vi "Set Poses.vi"(8 "error in (no error)":errorcluster, 10 "serial arm poses":T1[](array[typedef]), 11 "serial arm in":refnum<class "NI_Robotics_Serial Robot Arm.lvclass">) -> (0 "error out":errorcluster, 3 "serial arm out":refnum<class "NI_Robotics_Serial Robot Arm.lvclass">)   [LabVIEW 2017, in "NI_Robotics_Serial Robot Arm.lvclass"]
doc: "Sets the joint angles that make up <B>serial arm poses</B> you want to associate with a robotic arm."
uses:
  <vilib>/robotics/Kinematics/Robot/NI_Robotics_Serial Robot Arm.lvclass
  <vilib>/robotics/Kinematics/Robot/Robot Pose.ctl
  <vilib>/robotics/Kinematics/Robot/NI_Robotics_Serial Robot Arm.lvclass/NI_Robotics_Serial Robot Arm.ctl
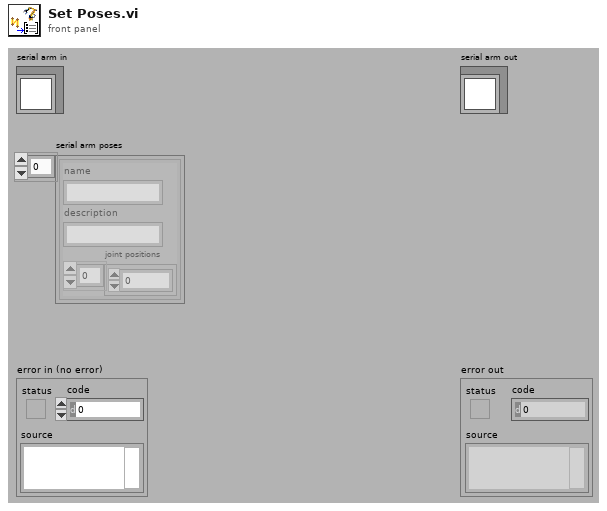
[diagram p1: front panel]
types:
  T1 = typedef "NI_Robotics_Serial Robot Arm.lvclass/Robot Pose.ctl" = cluster{"name":string, "description":string, "joint positions":dbl[]}
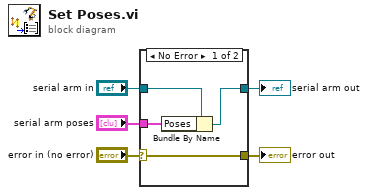
[diagram p0: block diagram]
diagram:
  n1 = case shown="No Error" "error in (no error)" {
    selector: "error in (no error)" -> [w9 w10]
    tunnel: [w9 w10] -> w4
    tunnel: [w7 w11] -> w2
    tunnel: "serial arm in" -> [w8 w11]
    tunnel: "serial arm poses" -> [w6 _]
    frame No Error {
      n2 = Bundle By Name(cluster=w8, "Poses"=w6) -> (w7:refnum<class "NI_Robotics_Serial Robot Arm.lvclass">)
    }
    frame Error {
    }
  }
  "error out" <- w4
  "serial arm out" <- w2
